vi "tcp_move_rel.vi"(6 "wait4motiondone":bool, 8 "error in (no error)":errorcluster, 9 "diff nm/u°":dbl, 10 "Axis":string(combo), 11 "IP address":string="172.16.6.101") -> (0 "error out":errorcluster, 2 "position":dbl, 3 "IP address out":string="172.16.6.101")   [LabVIEW 2012]
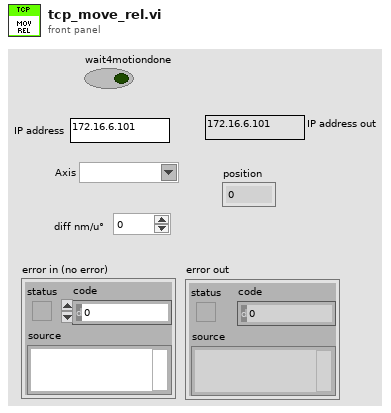
[diagram p1: front panel]
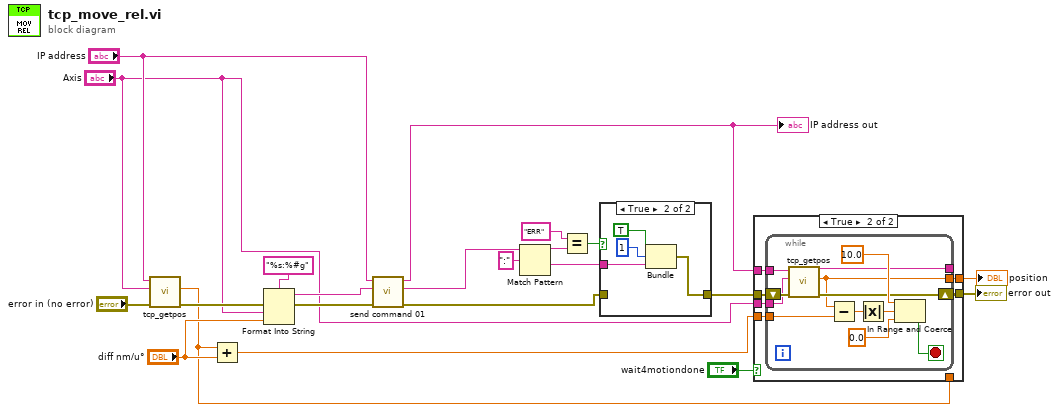
[diagram p0: block diagram]
diagram:
  n1 = call "tcp_getpos.vi"("error in (no error)"="error in (no error)", "Axis"="Axis", "IP address"="IP address") -> ("error out"=w11:errorcluster, "position"=w2:dbl)  [unwired: 6 in, 1 out]
  n2 = Add(x=w2, y="diff nm/u°") -> (x+y=w1:dbl)
  n3 = Format Into String(format string="%s:%#g", error in=w11, "Axis", "diff nm/u°") -> (resulting string=w21:string, error out=w10:errorcluster)  [unwired: 1 in]
  n4 = call "send command 01.vi"("error in (no error)"=w10, "command"=w21, "IP address in"="IP address") -> ("error out"=w14:errorcluster, "response"=w17:string, "IP address out"=w8:string)  [unwired: 6 in]
  "IP address out" <- w8
  n5 = Match Pattern(string=w17, regular expression=":") -> (before substring=w19:string, after substring=w15:string)  [unwired: 1 in, 2 out]
  n6 = Equal?(x="ERR", y=w19) -> (x = y?=w16:bool)
  n7 = case shown="True" w16 {
    tunnel: w15 -> [_ w25]
    tunnel: [w23 w24] -> w9
    tunnel: w14 -> [w23 _]
    frame False {
    }
    frame True {
      n8 = Bundle(TRUE, 1, "response"=w25) -> (w24:cluster{bool, i32, "response":string})  [unwired: 1 in]
    }
  }
  n9 = case shown="True" "wait4motiondone" {
    tunnel: w9 -> [w29 w35]
    tunnel: w1 -> [_ w34]
    tunnel: w8 -> [_ w33]
    tunnel: "Axis" -> [_ w32]
    tunnel: [w29 w31] -> w6
    tunnel: [w28 w30] -> w4
    tunnel: w2 -> [w28 _]
    frame False {
    }
    frame True {
      n10 = while {
        tunnel: w33 -> [w47]
        tunnel: w32 -> [w45]
        tunnel: w34 -> [w44]
        tunnel: [w37] -> _
        shift-right: [w38] -> w31
        shift-left: w35 -> [w46]
        tunnel: [w36] -> w30
        stop <- w39 stop-if-true
        n11 = call "tcp_getpos.vi"("error in (no error)"=w46, "Axis"=w45, "IP address"=w47) -> ("error out"=w38:errorcluster, "position"=w36:dbl, "IP address out"=w37:string)  [unwired: 6 in]
        n12 = Subtract(x=w36, y=w44) -> (x-y=w43:dbl)
        n13 = Absolute Value(x=w43) -> (abs(x)=w42:dbl)
        n14 = In Range and Coerce(upper limit=10.0, x=w42, lower limit=0.0) -> (In Range?=w39:bool)  [unwired: 1 out]
      }
    }
  }
  "error out" <- w6
  "position" <- w4
